vi "ToString.vi"(8 "error in (no error)":errorcluster, 11 "UnaryOperator in":refnum<class "UnaryOperator.lvclass">) -> (0 "error out":errorcluster, 2 "String":string, 3 "UnaryOperator out":refnum<class "UnaryOperator.lvclass">)   [LabVIEW 2019, in "Constraint.lvlib" / "UnaryOperator.lvclass"]
doc: "Returns a string representation of the object."
uses:
  UnaryOperator.lvclass
  Constraint/Constraint.lvclass
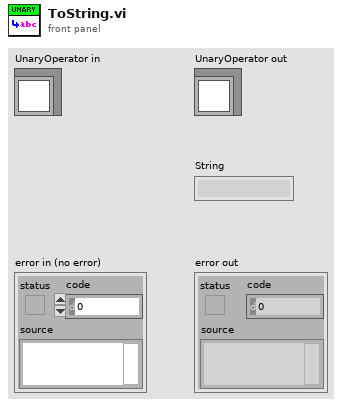
[diagram p1: front panel]
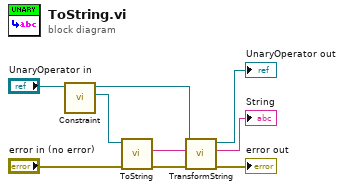
[diagram p0: block diagram]
diagram:
  n1 = call "Constraint.vi"("UnaryOperator in"="UnaryOperator in") -> ("Constraint.lvlib:Constraint.lvclass"=w1:refnum<class "Constraint.lvclass">, "UnaryOperator out"=w2:refnum<class "UnaryOperator.lvclass">)  [unwired: 9 in]
  n2 = call-dynamic "ToString.vi"("error in (no error)"="error in (no error)", "Constraint in"=w1) -> ("error out"=w9:errorcluster, "String"=w4:string)  [unwired: 7 in, 1 out]
  n3 = call-dynamic "TransformString.vi"("error in (no error)"=w9, "String"=w4, "UnaryOperator in"=w2) -> ("error out"=→"error out":errorcluster, "String out"=→"String":string, "UnaryOperator out"=→"UnaryOperator out":refnum<class "UnaryOperator.lvclass">)  [unwired: 6 in]
